vi "Pdash Style--constant.vi"() -> (3 "Style":T1={"Gris Obscuro Azul"=4079166, "Gris Medio Azul"=9343126, "Gris Claro Azul"=13817819, "Amarillo"=16763904, "Text color"=4079166, "Transparent"=4079166, "Fuente"="", "Text.Font:Size"=15})   [LabVIEW 2024]
uses:
  Pdash Style--cluster.ctl
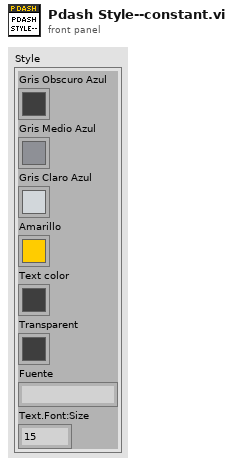
[diagram p1: front panel]
types:
  T1 = typedef "Pdash Style--cluster.ctl" = cluster{"Gris Obscuro Azul":u32, "Gris Medio Azul":u32, "Gris Claro Azul":u32, "Amarillo":u32, "Text color":u32, "Transparent":u32, "Fuente":string, "Text.Font:Size":u32}
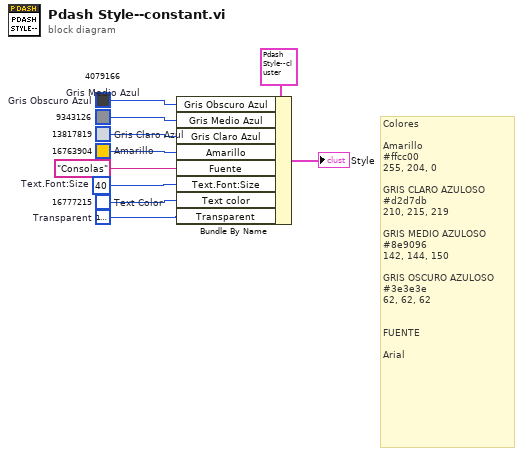
[diagram p0: block diagram]
diagram:
  w1 = u32 16777216  # Transparent
  w2 = u32 16777215  # Text Color
  w3 = u32 40  # Text.Font:Size
  w6 = u32 16763904  # Amarillo
  w7 = u32 13817819  # Gris Claro Azul
  w8 = u32 9343126  # Gris Medio Azul
  w9 = u32 4079166  # Gris Obscuro Azul
  # "Colores\n\nAmarillo\n#ffcc00\n255, 204, 0\n\nGRIS CLARO AZULOSO\n#d2d7db\n210, 215, 219\n\nGRIS MEDIO AZULOSO\n#8e9096\n142, 144, 150\n\nGRIS OSCURO AZULOSO\n#3e3e3e\n62, 62, 62\n\n\nFUENTE\n\nArial"
  n1 = Bundle By Name(cluster=T1 {"Gris Obscuro Azul"=4079166, "Gris Medio Azul"=9343126, "Gris Claro Azul"=13817819, "Amarillo"=16763904, "Text color"=4079166, "Transparent"=4079166, "Fuente"="", "Text.Font:Size"=15}, "Gris Obscuro Azul"=w9, "Gris Medio Azul"=w8, "Gris Claro Azul"=w7, "Amarillo"=w6, "Fuente"="Consolas", "Text.Font:Size"=w3, "Text color"=w2, "Transparent"=w1) -> (→"Style":T1)
